vi "DataHandle.vi"(6 "error IO":errorcluster, 8 "滑动杆":i16(slide) scale=3.5..18.0, 9 "地图":refnum<k7>(container) caption="网页浏览器", 10 "data":string, 11 "时间":timestamp) -> (0 "uid":i16, 1 "温度":sgl, 2 "经度显示":string, 3 "纬度显示":string, 4 "错误输出":errorcluster, 5 "储运信息簇":T1 {"记录时间" format="%<%H:%M:%S\n%Y/%m/%d>T"}, 7 "定位":bool)   [LabVIEW 2018]
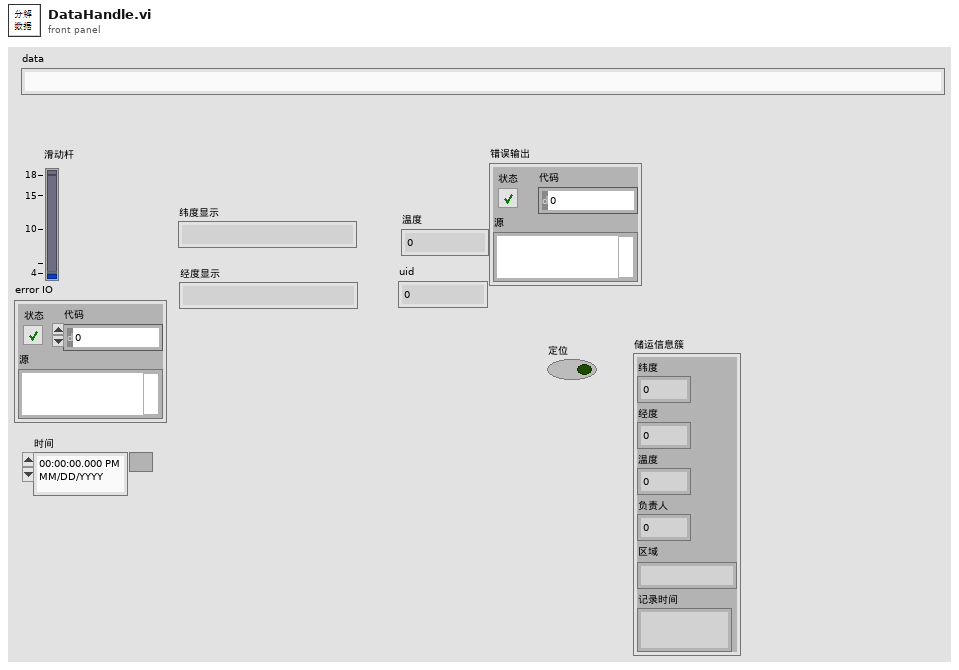
[diagram p1: front panel]
types:
  T1 = typedef "储运信息.ctl" = cluster{"纬度":sgl, "经度":sgl, "温度":sgl, "负责人":i32, "区域":string, "记录时间":timestamp}
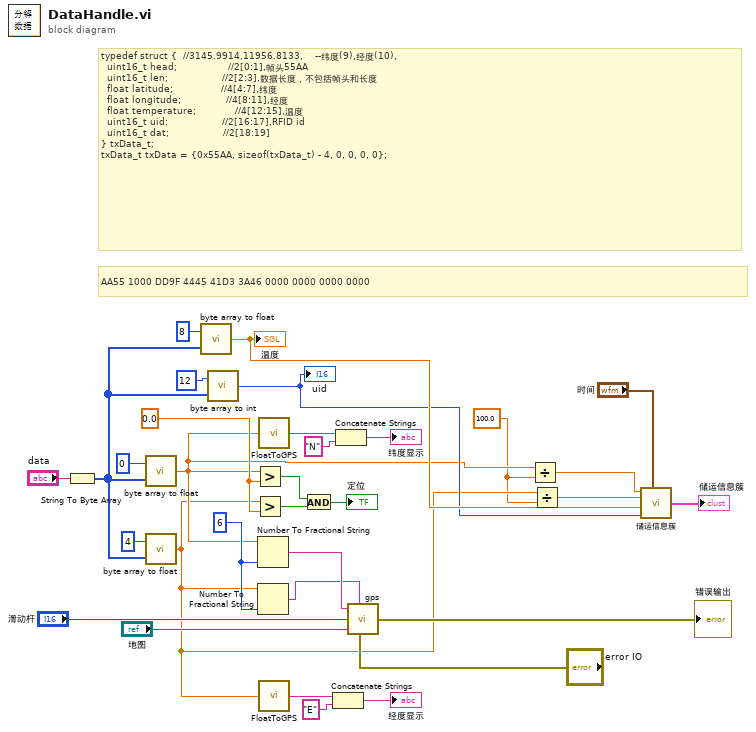
[diagram p0: block diagram]
diagram:
  w1 = 100.0
  w20 = i16 6 ("精度(6)")
  w32 = 0.0 ("y")
  # "AA55 1000 DD9F 4445 41D3 3A46 0000 0000 0000 0000"
  # "typedef struct {  //3145.9914,11956.8133,    --纬度(9),经度(10),\n  uint16_t head;                 //2[0:1],帧头55AA\n  uint16_t len;                  //2[2:3],数据长度，不包括帧头和长度\n  float latitude;                //4[4:7],纬度\n  float longitude;               //4[8:11],经度\n  float temperature;             //4[12:15],温度\n  uint16_t uid;                  //2[16:17],RFID id\n  uint16_t dat;                  //2[18:19]\n} txData_t;\ntxData_t txData = {0x55AA, sizeof(txData_t) - 4, 0, 0, 0, 0};"
  n1 = String To Byte Array(string="data") -> (unsigned byte array=w25:u8[])
  n2 = call "byte array to float.vi"("unsigned byte array"=w25, "索引"=0) -> ("数值"=w5:sgl)
  n3 = call "byte array to float.vi"("unsigned byte array"=w25, "索引"=4) -> ("数值"=w3:sgl)
  n4 = call "byte array to float.vi"("unsigned byte array"=w25, "索引"=8) -> ("数值"=w9:sgl)
  "温度" <- w9
  n5 = call "byte array to int.vi"("unsigned byte array"=w25, "索引"=12) -> ("数值"=w8:i16)
  "uid" <- w8
  n6 = Greater?(x=w5, y=w32) -> (0:w29:bool)
  n7 = Greater?(x=w3, y=w32) -> (0:w30:bool)
  n8 = Number To Fractional String(number=w5, precision (6)=w20) -> (F-format string=w13:string)  [unwired: 2 in]
  n9 = Number To Fractional String(number=w3, precision (6)=w20) -> (F-format string=w12:string)  [unwired: 2 in]
  n10 = call "FloatToGPS.vi"("数字"=w5) -> ("string"=w21:string)
  n11 = call "FloatToGPS.vi"("数字"=w3) -> ("string"=w19:string)
  n12 = And(x=w29, y=w30) -> (x .and. y?=→"定位":bool)
  n13 = Concatenate Strings(w19, "E" ("字符串")) -> (→"经度显示":string)
  n14 = Concatenate Strings(w21, "N" ("字符串")) -> (→"纬度显示":string)
  n15 = call "gps.vi"("纬度"=w13, "经度"=w12, "滑动杆"="滑动杆", "地图"="地图", "error IO"="error IO") -> ("错误输出"=→"错误输出":errorcluster)
  n16 = Divide(x=w5, y=w1) -> (x/y=w4:dbl)
  n17 = Divide(x=w3, y=w1) -> (x/y=w2:dbl)
  n18 = call "储运信息簇.vi"("纬度"=w4, "经度"=w2, "温度"=w9, "编号"=w8, "时间"="时间") -> ("待写入的簇"=→"储运信息簇":T1)
